vi "probe_point_names.vi"() -> (2 "Names":string[](array[string]))   [LabVIEW 2013]
uses:
  probe_point.ctl
panel:
  out "Probe point dummy":T1
  # "Return an array of strings naming the probe points.\nAs of LV 2010 SP1, there were some interactions with\nthe execution properties for what we do here to work\n(getting a property from the control)  In particular, \nit seems that this VI can't be reentrant."
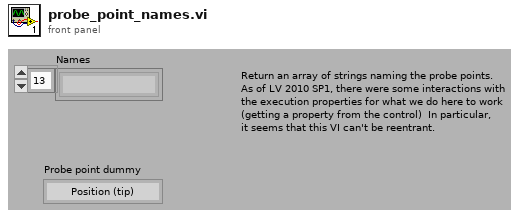
[diagram p1: front panel]
types:
  T1 = typedef "probe_point.ctl" = enum16{"Position (tip)", "Position (RCM)", "Null pos (tip)", "Null pos (RCM)", "V limiter (tip)", "V Limiter (RCM)", "Goal (tip)", "Goal (RCM)", "Link pos 0", "Link pos 1", "KF link pos 0", "KF link pos 1", "Link rate 0", "Link rate 1", "Link residue 0", "Link residue 1", "Link goal 0", "Link goal 1", "Rate limit 0", "Rate limit 1", "Link error 0", "Link error 1", "Controller 0", "Controller 1", "Output 0", "Output 1", "Drive 0", "Drive 1", "Stimulus 0", "Stimulus 1", "Trace data 0", "Trace data 1", "Analog data 0", "Analog data 1", "Status flags", "Light 0", "Light 1", "Light 2", "Light 3", "Light 4", "Light 5", "Goal origin", "Goal rotation 0", "Goal rotation 1", "Goal rotation 2", "Output origin", "Output rotation 0", "Output rotation 1", "Output rotation 2", "Handle origin", "Handle rotation 0", "Handle rotation 1", "Handle rotation 2", "Handle position", "Handle velocity", "Handle acceleration", "Handle angles", "Handle angle rates", "Handle pos residue", "Handle angle residue", "Trace length"}
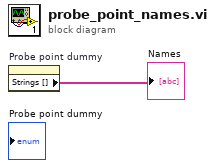
[diagram p0: block diagram]
diagram:
  n1 = property on="Probe point dummy" class="Enum (strict)"() -> ("Strings []"=→"Names":string[])  [unwired: 2 in, 2 out]
